vi "22Pixel.vi"() -> ()   [LabVIEW 2009, in "menu item.lvclass"]
uses:
  menu item.lvclass
panel:
  out "22 pixel":u32
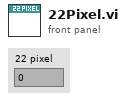
[diagram p1: front panel]
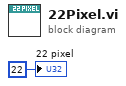
[diagram p0: block diagram]
diagram:
  "22 pixel" <- u32 22 ("1 pixel")
